vi "Read Chip ID.vi"(7 "SlaveID":u8, 8 "error in (no error)":errorcluster, 11 ".NET Refnum in":refnum<k24>) -> (0 "error out":errorcluster, 2 "ReadInputRegisters":u16[](array[numeric]), 3 ".NET Refnum out":refnum<k24>)   [LabVIEW 2013]
uses:
  C:/Users/User/Desktop/Modbus Demo/DLL/Modbus.dll
  DLL/Modbus.dll
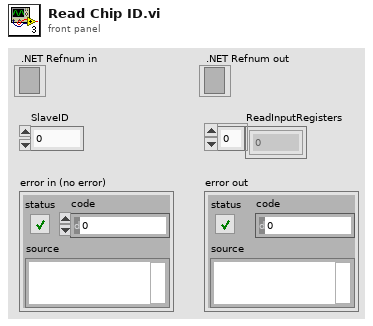
[diagram p1: front panel]
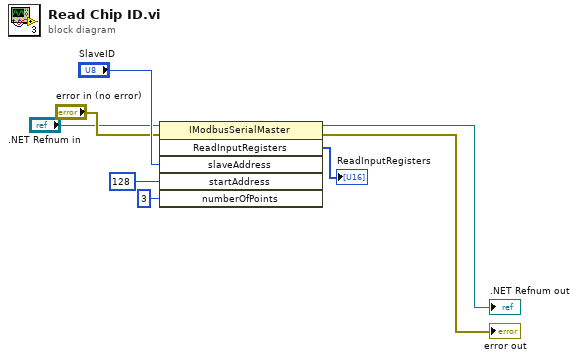
[diagram p0: block diagram]
diagram:
  n1 = invoke class="IModbusSerialMaster" method="ReadInputRegisters"(reference=".NET Refnum in", error in="error in (no error)", "slaveAddress"="SlaveID", "startAddress"=u16 128, "numberOfPoints"=u16 3) -> (reference out=→".NET Refnum out":refnum<k24>, error out=→"error out":errorcluster, "ReadInputRegisters"=→"ReadInputRegisters":u16[])  [unwired: 1 in, 3 out]
